vi "CU_readClassifierParams.vi"(8 "error in (no error)":errorcluster, 11 "ClassifierClass in":refnum<class "ClassifierClass.lvclass">) -> (0 "error out":errorcluster, 1 "Classifier Metaparameter out":dbl, 2 "ClassifierType out":T1=enum."k NN Classifier", 3 "ClassifierClass out":refnum<class "ClassifierClass.lvclass">)   [LabVIEW 2016, in "Classifier.lvlib" / "ClassifierClass.lvclass"]
uses:
  ClassifierClass.lvclass
  CU_ClassifierTypes.ctl
  ClassifierClass.lvclass/ClassifierClass.ctl
  Classifier.lvlib
panel:
  # "This VI is a part of BCI Design library, http://www.ru-bci.org \nCopyright © 2020, Sotnikov Peter, All rights reserved. License: GNU GPLv3"
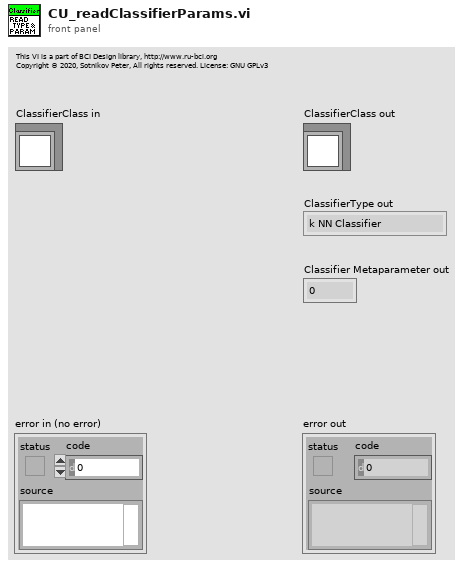
[diagram p1: front panel]
types:
  T1 = typedef "Classifier.lvlib/CU_ClassifierTypes.ctl" = enum16{"Multilayer perceptron", "k NN Classifier", "SVM Committee", "Mahalanobis distance", "SVM Classifier"}
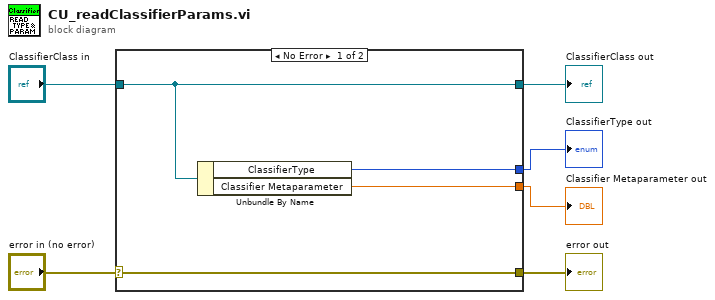
[diagram p0: block diagram]
diagram:
  n1 = case shown="No Error" "error in (no error)" {
    selector: "error in (no error)" -> [w10 w11]
    tunnel: [w10 w11] -> w5
    tunnel: [w9 w12] -> w3
    tunnel: "ClassifierClass in" -> [w9 w12]
    tunnel: [w8 _] -> w2
    tunnel: [w7 _] -> w1
    frame No Error {
      n2 = Unbundle By Name(w9) -> ("ClassifierType"=w8:T1, "Classifier Metaparameter"=w7:dbl)
    }
    frame Error {
    }
  }
  "error out" <- w5
  "ClassifierClass out" <- w3
  "ClassifierType out" <- w2
  "Classifier Metaparameter out" <- w1
